vi "Initialize.vi"(8 "error in (no error)":errorcluster, 11 "Masterflex Settings in":T1={"VISA resource name"="", "Simulated?"=FALSE, "Pump Number"=1.0, "Reverse?"=FALSE} {"Pump Number" min=1.0 max=20.0 step=1.0}) -> (0 "error out":errorcluster, 1 "Initialized":bool, 2 "No Pump Connected":bool, 3 "Masterflex Settings out":T1={"VISA resource name"="", "Simulated?"=FALSE, "Pump Number"=1.0, "Reverse?"=FALSE} {"Pump Number" min=1.0 max=20.0 step=1.0})   [LabVIEW 2018, in "Masterflex 7550-30.lvlib"]
uses:
  Masterflex 7550-30.lvlib
  Controls/Settings Cluster.ctl
  <vilib>/Instr/_visa.llb/VISA Configure Serial Port (Instr).vi
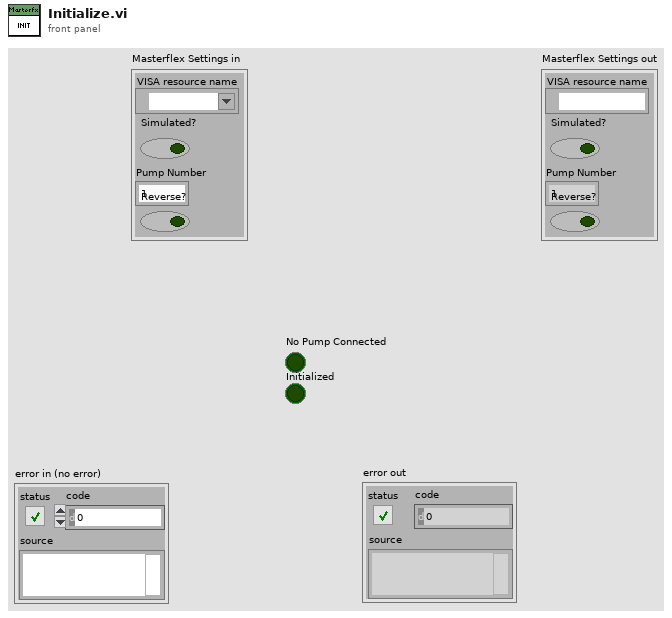
[diagram p1: front panel]
types:
  T1 = typedef "Masterflex 7550-30.lvlib/Settings Cluster.ctl" = cluster{"VISA resource name":refnum<visa-resource-name>, "Simulated?":bool, "Pump Number":dbl, "Reverse?":bool}
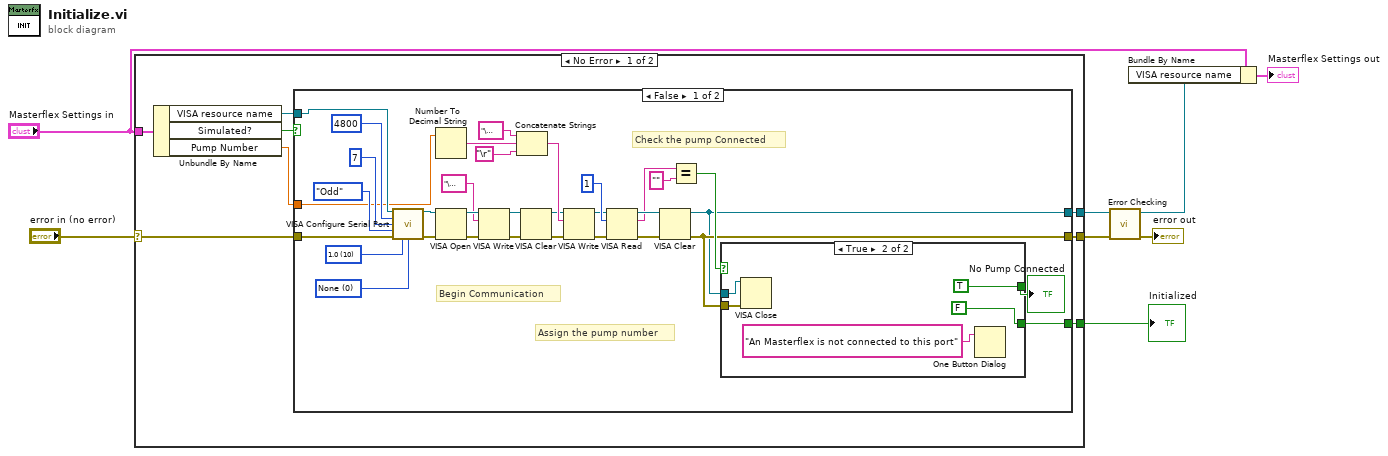
[diagram p0: block diagram]
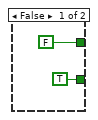
[diagram p2: hidden frame]
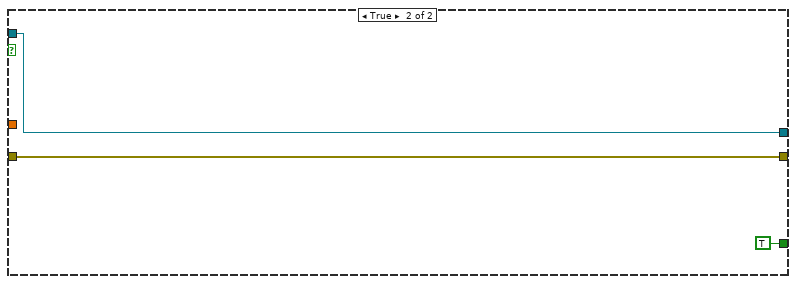
[diagram p3: hidden frame]
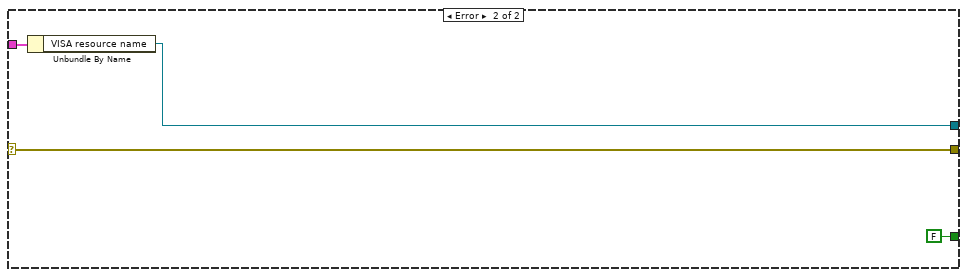
[diagram p4: hidden frame]
diagram:
  n1 = case shown="No Error" "error in (no error)" {
    selector: "error in (no error)" -> [w16 w63]
    tunnel: "Masterflex Settings in" -> [w11 w62]
    tunnel: [w12 w63] -> w5
    tunnel: [w10 w61] -> w2
    tunnel: [w9 FALSE] -> w1
    frame No Error {
      n2 = Unbundle By Name(w11) -> ("VISA resource name"=w14:refnum<visa-resource-name>, "Simulated?"=w15:bool, "Pump Number"=w13:dbl)
      n3 = case shown="False" w15 {
        tunnel: w16 -> [w43 w59]
        tunnel: w14 -> [w41 w58]
        tunnel: w13 -> [w33 _]
        tunnel: [w20 w59] -> w12
        tunnel: [w19 w58] -> w10
        tunnel: [w17 TRUE] -> w9
        frame False {
          w45 = u16 0 items=["None", "XON/XOFF", "RTS/CTS", "XON/XOFF & RTS/CTS", "DTR/DSR", "XON/XOFF & DTR/DSR"] ("flow control (0:none)")
          w46 = u16 10 items=["1.0"=10, "1.5"=15, "2.0"=20] ("stop bits (10: 1 bit)")
          # "Check the pump Connected"
          # "Assign the pump number"
          # "Begin Communication"
          n4 = call-poly "VISA Configure Serial Port"("VISA resource name"=w41, "baud rate (9600)"=u32 4800, "data bits (8)"=u16 7, "parity (0:none)"=enum16{"None", "Odd", "Even", "Mark", "Space"}."Odd", "error in (no error)"=w43, "stop bits (10: 1 bit)"=w46, "flow control (0:none)"=w45) -> ("VISA resource name out"=w42:refnum<visa-resource-name>, "error out"=w44:errorcluster)  [unwired: 7 in]
          n5 = Number To Decimal String(number=w33) -> (decimal integer string=w34:string)  [unwired: 1 in]
          n6 = VISA Open(error in (no error)=w44, VISA resource name=w42) -> (VISA resource name=w40:refnum<visa-resource-name>, error out=w39:errorcluster)  [unwired: 3 in]
          n7 = VISA Write(VISA resource name=w40, write buffer="\u0005", error in (no error)=w39) -> (VISA resource name out=w29:refnum<visa-resource-name>, error out=w28:errorcluster)  [unwired: 1 out]
          n8 = Concatenate Strings("\u0002" ("string"), w34, "\r") -> (w35:string)
          n9 = VISA Clear(VISA resource name=w29, error in (no error)=w28) -> (VISA resource name out=w27:refnum<visa-resource-name>, error out=w26:errorcluster)
          n10 = VISA Write(VISA resource name=w27, write buffer=w35, error in (no error)=w26) -> (VISA resource name out=w31:refnum<visa-resource-name>, error out=w30:errorcluster)  [unwired: 1 out]
          n11 = VISA Read(VISA resource name=w31, byte count=u32 1, error in (no error)=w30) -> (VISA resource name out=w23:refnum<visa-resource-name>, read buffer=w21:string, error out=w24:errorcluster)  [unwired: 1 out]
          n12 = VISA Clear(VISA resource name=w23, error in (no error)=w24) -> (VISA resource name out=w19:refnum<visa-resource-name>, error out=w20:errorcluster)
          n13 = Equal?(x=w21, y="") -> (x = y?=w25:bool)
          n14 = case shown="True" w25 {
            tunnel: w19 -> [_ w55]
            tunnel: w20 -> [_ w54]
            tunnel: [FALSE TRUE] -> w18
            tunnel: [TRUE FALSE] -> w17
            frame False {
            }
            frame True {
              n15 = VISA Close(VISA resource name=w55, error in (no error)=w54) -> ()  [unwired: 1 out]
              n16 = One Button Dialog(message="An Masterflex is not connected to this port") -> ()  [unwired: 1 in, 1 out]
            }
          }
          "No Pump Connected" <- w18
        }
        frame True {
        }
      }
    }
    frame Error {
      n17 = Unbundle By Name(w62) -> ("VISA resource name"=w61:refnum<visa-resource-name>)
    }
  }
  "Initialized" <- w1
  n18 = call "Error Checking.vi"("error in (no error)"=w5, "VISA resource name"=w2) -> ("error out"=→"error out":errorcluster, "VISA resource name"=w7:refnum<visa-resource-name>)  [unwired: 7 in, 1 out]
  n19 = Bundle By Name(cluster="Masterflex Settings in", "VISA resource name"=w7) -> (→"Masterflex Settings out":T1)
